vi "Create Formatter.vi"(8 "error in":errorcluster, 9 "Format Specifier":string="%s - %-8s - %s - %s - %d - %s", 10 "Datetime format":string="%.;%Y-%m-%d %H:%M:%S%3u") -> (0 "error out":errorcluster, 3 "Formatter out":refnum<class "Formatter.lvclass">)   [LabVIEW 2024, in "hse-logger.lvlib" / "Formatter.lvclass"]
doc: "Creates a default Formatter object with a default format string and datetime string in ISO format with milliseconds.\n\nInputs of the Format Into String node are:\n---------------------------------------------\n 1. Date Time (formatted by the \"Datetime Format\" string)\n 2. Log Level\n 3. Log Message\n 4. Call Chain\n 5. Error Code\n 6. Error Source\n\n____\nHAMPEL SOFTWARE ENGINEERING v2.2.2 (2025-01-16 15:41)"
uses:
  <vilib>/Hampel Software Engineering/HSE Logger/Formatter/Formatter.lvclass
panel:
  # "Time - Level - Callchain - Message - Error Code - Error Message"
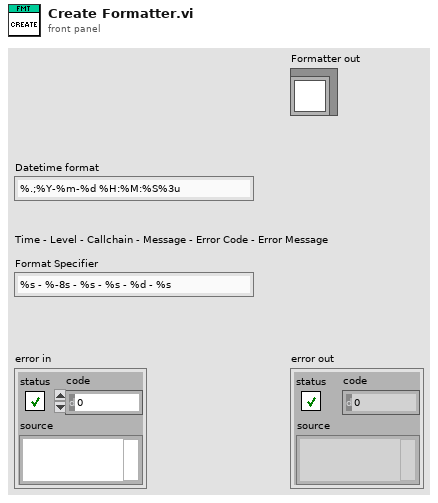
[diagram p1: front panel]
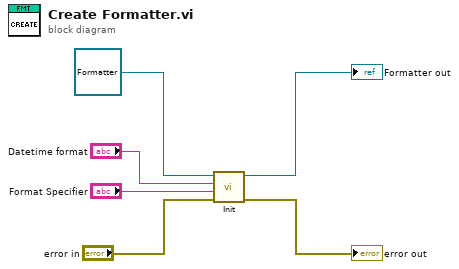
[diagram p0: block diagram]
diagram:
  n1 = call-dynamic "Init.vi"("error in"="error in", "Format Specifier"="Format Specifier", "Datetime format"="Datetime format", "Formatter in"=refnum<class "Formatter.lvclass"> refnum) -> ("error out"=→"error out":errorcluster, "Formatter out"=→"Formatter out":refnum<class "Formatter.lvclass">)  [unwired: 6 in]
